vi "PIDAutoTune_Step.vi"(5 "Procedure Type":enum16{"Open Loop Step", "Closed Loop Step"}(ring), 7 "Configuration Parameters":T2={"Controller Constant Type"=enum."Ziegler Nicols - Normal", "Type of Controller"=enum."PI", "CO Offset"=0.25, "Kn"=1.0, "Tuning Tolerance"=0.001, "Plant Tolerance"=0.001, "Newest Avg Time "=1, "Long Ave Time"=6}, 8 "Sampling Time dt (s)":dbl=0.02, 9 "Tune":bool, 10 "Measurement  (PV)":dbl, 11 "Control Output (Co)":dbl) -> (0 "Plant and Test Data":T4, 1 "New Tuning Parameters":T3, 2 "Tuning Done":bool, 3 "Adj CO":dbl, 4 "Error Occured":bool, 6 "Diagnostic Info":T1)   [LabVIEW 2019, in "Trajectory_Library.lvlib"]
uses:
  Timer_New.vi
  LinearFilter_ResetToValue.vi
  LinearFilter_Calculate.vi
  <vilib>/Utility/semaphor.llb/Obtain Semaphore Reference.vi
  Timer_Reset.vi
  Timer_Start.vi
  Timer_Stop.vi
  Timer_HasPeriodPassedOnce.vi
  LinearFilter_MovingAverage.vi
  LinearFilter_LowPassBW1.vi
  LinearFilter_LowPassBW2.vi
  LinearFilter_HighPassBW1.vi
  LinearFilter_HighPassBW2.vi
  Trajectory_Library.lvlib
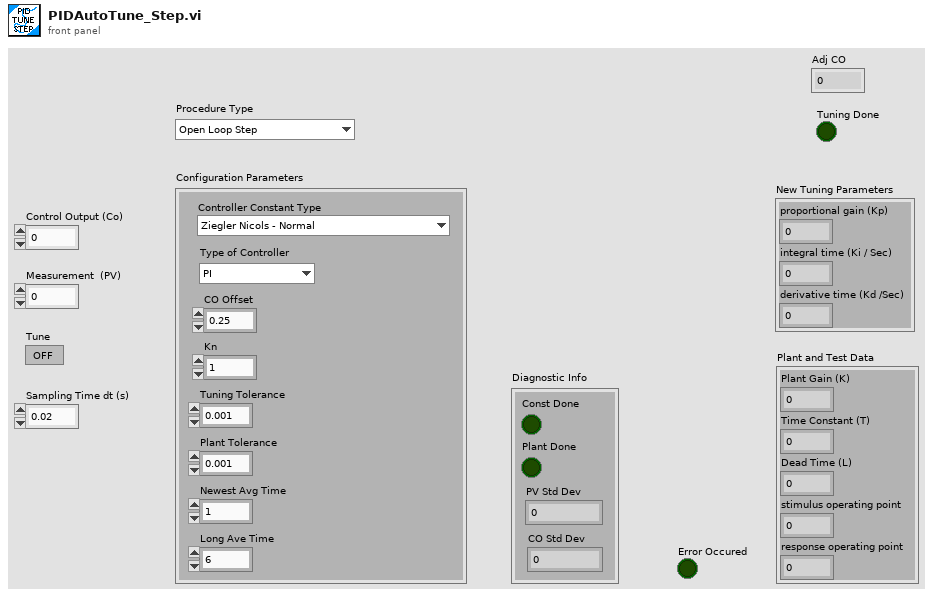
[diagram p1: front panel]
types:
  T1 = cluster{"Const Done":bool, "Plant Done":bool, "PV Std Dev":dbl, "CO Std Dev":dbl}
  T2 = cluster{"Controller Constant Type":enum16{"Ziegler Nicols - Fast", "Ziegler Nicols - Normal", "Ziegler Nicols - Slow", "CHR regulator - 0% overshoot", "CHR regulator - 20% overshoot", "CHR servo - 0 % overshoot", "CHR servo - 20% overshoot"}, "Type of Controller":enum16{"P", "PI", "PID"}, "CO Offset":dbl, "Kn":dbl, "Tuning Tolerance":dbl, "Plant Tolerance":dbl, "Newest Avg Time ":i32, "Long Ave Time":i32}
  T3 = cluster{"proportional gain (Kp)":dbl, "integral time (Ki / Sec)":dbl, "derivative time (Kd /Sec)":dbl}
  T4 = cluster{"Plant Gain (K)":dbl, "Time Constant (T)":dbl, "Dead Time (L)":dbl, "stimulus operating point":dbl, "response operating point":dbl}
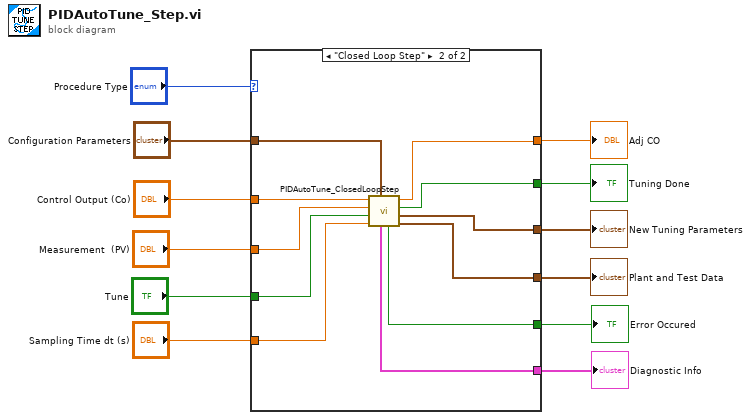
[diagram p0: block diagram]
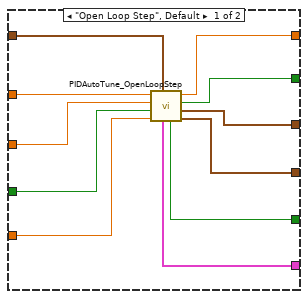
[diagram p2: hidden frame]
diagram:
  n1 = case shown="\"Closed Loop Step\"" "Procedure Type" {
    tunnel: "Configuration Parameters" -> [w23 w34]
    tunnel: "Control Output (Co)" -> [w22 w33]
    tunnel: "Measurement  (PV)" -> [w21 w32]
    tunnel: "Tune" -> [w20 w31]
    tunnel: "Sampling Time dt (s)" -> [w19 w30]
    tunnel: [w18 w29] -> w6
    tunnel: [w17 w28] -> w5
    tunnel: [w16 w27] -> w4
    tunnel: [w15 w26] -> w3
    tunnel: [w14 w25] -> w2
    tunnel: [w13 w24] -> w1
    frame "Open Loop Step", Default {
      n2 = call "PIDAutoTune_OpenLoopStep.vi"("Tuning Parameters"=w23, "Sampling Time dt (s)"=w19, "Tune"=w20, "Measurement  (PV)"=w21, "Control Output (Co)"=w22) -> ("Plant and Test Data"=w15:T4, "New Tuning Parameters"=w16:T3, "Tuning Done"=w17:bool, "Adj CO"=w18:dbl, "Error Occured"=w14:bool, "Diagnostic"=w13:T1)  [unwired: 1 in]
    }
    frame "Closed Loop Step" {
      n3 = call "PIDAutoTune_ClosedLoopStep.vi"("Tuning Parameters"=w34, "Sampling Time dt (s)"=w30, "Tune"=w31, "Measurement  (PV)"=w32, "Control Output (Co)"=w33) -> ("Plant and Test Data"=w26:T4, "New Tuning Parameters"=w27:T3, "Tuning Done"=w28:bool, "Adj CO"=w29:dbl, "Error Occured"=w25:bool, "Diagnostic"=w24:T1)  [unwired: 1 in]
    }
  }
  "Plant and Test Data" <- w3
  "Tuning Done" <- w5
  "Adj CO" <- w6
  "New Tuning Parameters" <- w4
  "Error Occured" <- w2
  "Diagnostic Info" <- w1
